vi "top VI.vi"() -> ()   [LabVIEW 2014]
panel:
  in  "stop":bool
  in  "OK Button 3":bool
  in  "OK Button 2":bool
  in  "OK Button":bool
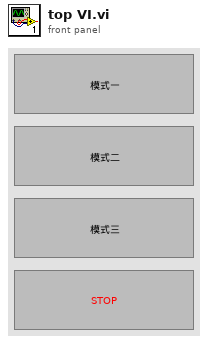
[diagram p1: front panel]
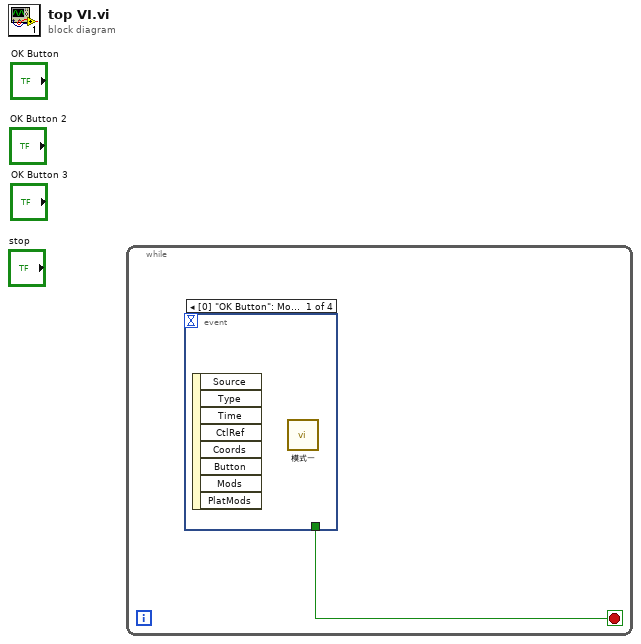
[diagram p0: block diagram]
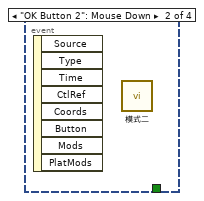
[diagram p2: hidden frame]
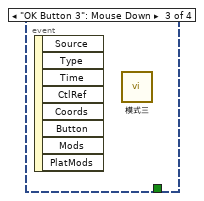
[diagram p3: hidden frame]
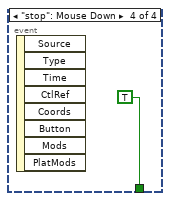
[diagram p4: hidden frame]
diagram:
  n1 = while {
    stop <- w1 stop-if-true
    n2 = event shown="[0] \"OK Button\": Mouse Down" {
      selector: _ -> [_ _ _ _]
      dyn-events: _ -> [_ _ _ _]
      timeout: _ -> [_ _ _ _]
      tunnel: [_ _ _ TRUE] -> w1
      event "OK Button": Mouse Down {
        n3 = event-data() -> ()  [unwired: 1 in, 8 out]
        n4 = call "模式一.vi"() -> ()  [unwired: 12 in]
      }
      event "OK Button 2": Mouse Down {
        n5 = event-data() -> ()  [unwired: 1 in, 8 out]
        n6 = call "模式二.vi"() -> ()  [unwired: 12 in]
      }
      event "OK Button 3": Mouse Down {
        n7 = event-data() -> ()  [unwired: 1 in, 8 out]
        n8 = call "模式三.vi"() -> ()  [unwired: 12 in]
      }
      event "stop": Mouse Down {
        n9 = event-data() -> ()  [unwired: 1 in, 8 out]
      }
    }
  }
